vi "Namen in der Gasliste aendern.vi"(11 "Messbereich":u16) -> ()   [LabVIEW 2020, in "Messdaten.lvlib"]
uses:
  Messdaten.lvlib
  Seiten/FT-IR/FGV FT-IR Gasliste Aktionen.ctl
  Aktionen FGV Messdaten.ctl
  Seiten/FT-IR/FT-IR.lvlib
  Seiten/Log Konfig/LogKonfig.lvlib
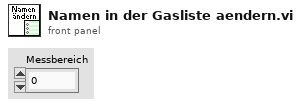
[diagram p1: front panel]
types:
  T1 = typedef "FT-IR.lvlib/FGV FT-IR Gasliste Aktionen.ctl" = enum16{"lesen", "Gasliste FT-IR", "Gasliste ausgelesen", "laden", "speichern", "löschen"}
  T2 = typedef "Messdaten.lvlib/Aktionen FGV Messdaten.ctl" = enum16{"lesen", "schreiben", "löschen", "Mittelwerte", "Komponente"}
  T3 = typedef "String - Ausgabefeld.ctl" = string
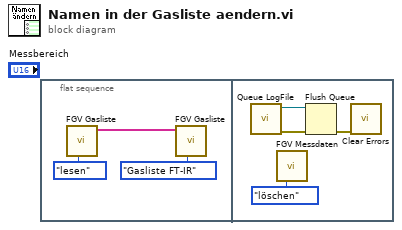
[diagram p0: block diagram]
diagram:
  n1 = flat-sequence {
    frame #0 {
      n2 = call "FGV Gasliste.vi"("Aktionen"=FGV_FT-IR_Gasliste_Aktionen."lesen") -> ("Aktuelle Gasliste FT-IR"=w1:T3[])  [unwired: 8 in, 2 out]
      n3 = call "FGV Gasliste.vi"("Aktionen"=FGV_FT-IR_Gasliste_Aktionen."Gasliste FT-IR", "Aktuelle Gasliste FT-IR"=w1) -> ()  [unwired: 7 in, 3 out]
    }
    frame #1 {
      n4 = call "Queue LogFile.vi"() -> ("error out"=w7:errorcluster, "Queue (Ausgang)"=w6:refnum<queue>)  [unwired: 6 in]
      n5 = call "FGV Messdaten.vi"("Aktionen"=Aktionen_FGV_Messdaten."löschen") -> ()  [unwired: 6 in, 9 out]
      n6 = Flush Queue(queue=w6, error in (no error)=w7) -> (error out=w4:errorcluster)  [unwired: 2 out]
      n7 = call <vilib>:"Clear Errors.vi"("error in (no error)"=w4) -> ()  [unwired: 5 in, 2 out]
    }
  }
